vi "Example Graph - Weight Callback.vi"(4 "Weight":refnum<user-event>, 5 "Event Data":cluster{"sender":refnum<k24>, "weight":i32}, 6 "Control Ref":refnum<k24>, 7 "Event Common Data":T1) -> ()   [LabVIEW 2010]
uses:
  C:/tf/play/labview/Tinkerforge.dll
  Tinkerforge.dll
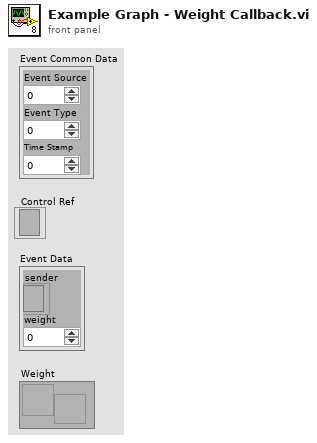
[diagram p1: front panel]
types:
  T1 = cluster{"Event Source":i32, "Event Type":u32, "Time Stamp":u32}
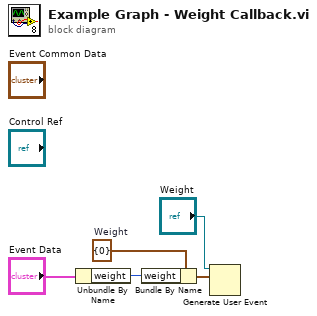
[diagram p0: block diagram]
diagram:
  w3 = cluster{"weight":i32} {"weight"=0}  # Weight
  n1 = Unbundle By Name("Event Data") -> ("weight"=w4:i32)
  n2 = Bundle By Name(cluster=w3, "weight"=w4) -> (w2:cluster{"weight":i32})
  n3 = Generate User Event(user event="Weight", event data cluster=w2) -> ()  [unwired: 1 in, 2 out]
